vi "Show Panel.vi"(8 "error in (no error)":errorcluster, 11 "View In":refnum<class "View.lvclass">) -> (0 "error out":errorcluster, 3 "View Out":refnum<class "View.lvclass">)   [LabVIEW 2020, in "View.lvclass"]
doc: "Show the front panel of the View."
uses:
  View.lvclass
  C:/git/astemes-triarc-framework/source/Framework/Process/Process.lvclass
  Process/Public/Lifecycle/API Mode.ctl
  Process/Process.lvclass/Process.ctl
  Process/Private/SubVIs/Handle Debug Data.vi
  Logging/Log Debug.vi
  <vilib>/AdvancedString/1D String Array to Delimited String.vi
  <vilib>/Utility/High Resolution Relative Seconds.vi
  <vilib>/Utility/error.llb/Error Cluster From Error Code.vi
  Process/Public/Read Name.vi
  <vilib>/ErrorRing/Error Ring.xnode
  Callback/Callback.lvclass
  Process/Process.lvclass
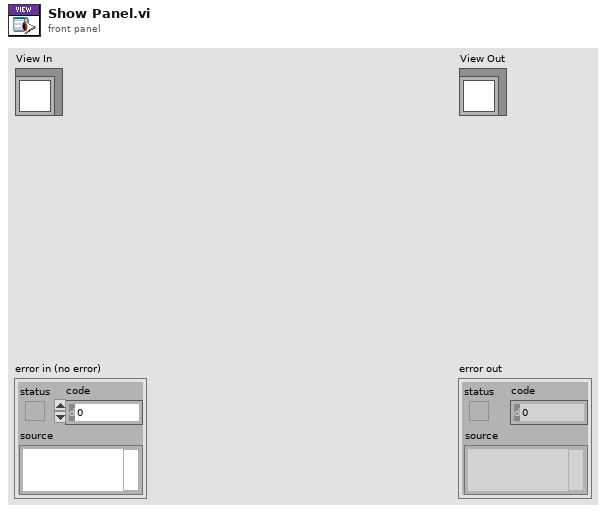
[diagram p1: front panel]
types:
  T1 = typedef "Process.lvclass/API Mode.ctl" = enum16{"Send Message", "Handle Message"}
  T2 = typedef "Process.lvclass/Lifecycle State.ctl" = enum16{"Uninitialized", "Initialized", "Started", "Running", "Stopped", "Finished"}
  T3 = enum32{"Invalid", "Standard", "Closed", "Hidden", "Minimized", "Maximized"}
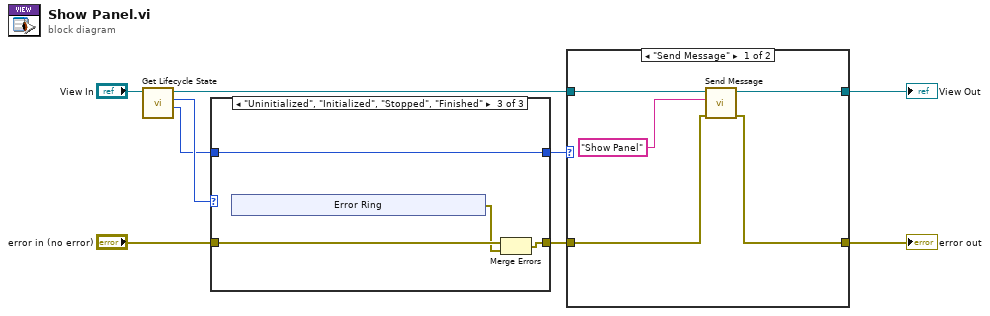
[diagram p0: block diagram]
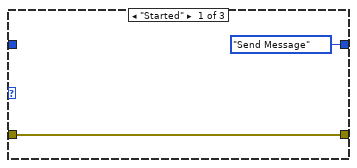
[diagram p2: hidden frame]
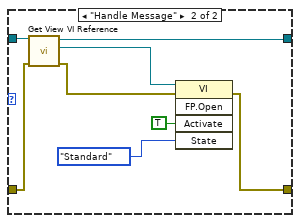
[diagram p4: hidden frame]
diagram:
  n1 = call "Get Lifecycle State.vi"("Process In"="View In") -> ("API Mode"=w1:T1, "Lifecycle State"=w5:T2, "Process Out"=w6:refnum<class "View.lvclass">)  [unwired: 7 in, 1 out]
  n2 = case shown="\"Uninitialized\", \"Initialized\", \"Stopped\", \"Finished\"" w5 {
    tunnel: [w11 w13 w16] -> w4
    tunnel: "error in (no error)" -> [w11 w13 w17]
    tunnel: w1 -> [_ w12 w14]
    tunnel: [API_Mode."Send Message" ("API Mode") w12 w14] -> w2
    frame "Started" {
    }
    frame "Running" {
    }
    frame "Uninitialized", "Initialized", "Stopped", "Finished" {
      n3 = xnode "Error Ring"() -> ("error out"=w15:errorcluster)
      n4 = Merge Errors(w17, w15) -> (w16:errorcluster)
    }
  }
  n5 = case shown="\"Send Message\"" w2 {
    tunnel: [w26 w29] -> w8
    tunnel: [w25 w27] -> w7
    tunnel: w4 -> [w24 w28]
    tunnel: w6 -> [w22 w30]
    frame "Send Message" {
      n6 = call "Send Message.vi"("error in (no error)"=w24, "Message"="Show Panel", "Process In"=w22) -> ("error out"=w25:errorcluster, "Process Out"=w26:refnum<class "View.lvclass">)  [unwired: 7 in]
    }
    frame "Handle Message" {
      n7 = call "Get View VI Reference.vi"("error in (no error)"=w28, "View In"=w30) -> ("error out"=w31:errorcluster, "View VI Reference"=w34:refnum<vi>, "View Out"=w29:refnum<class "View.lvclass">)  [unwired: 7 in]
      n8 = invoke class="VI" method="FP.Open"(reference=w34, error in=w31, "Activate"=TRUE ("Activate?"), "State"=T3."Standard") -> (error out=w27:errorcluster)  [unwired: 1 in, 4 out]
    }
  }
  "error out" <- w7
  "View Out" <- w8
